vi "TupnOn.vi"(8 "error in (no error)":errorcluster, 11 "Pump_1AI_1DO_2DI in":refnum<class "Engine_1DO_2DI.lvclass">) -> (0 "error out":errorcluster, 3 "Pump_1AI_1DO_2DI out":refnum<class "Engine_1DO_2DI.lvclass">)   [LabVIEW 2019, in "Engine_1DO_2DI.lvclass"]
uses:
  Engine_1DO_2DI.lvclass
  C:/Users/H4001/Documents/GitHub/H4000/src/Device_class/Device.lvclass
  Engine_1DO_2DI.lvclass/Engine_1DO_2DI.ctl
  Device_class/Device.lvclass/Device.ctl
  TypeDef/State Engine.ctl
  FPGA_API_class/FPGA API.lvclass
  Device_class/Device.lvclass
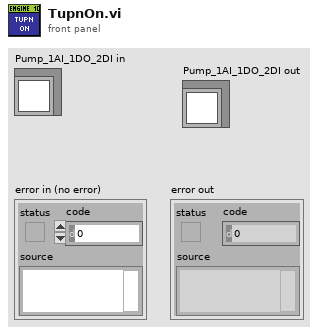
[diagram p1: front panel]
types:
  T1 = typedef "State Engine.ctl" = enum16{"Unknown", "Off", "TupningOn", "On", "TurningOff"}
  T2 = typedef "DO index.ctl" = u8
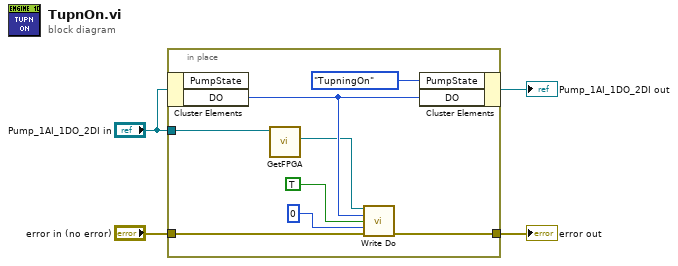
[diagram p0: block diagram]
diagram:
  n1 = in-place {
    in-place-border: [w8] -> w3
    in-place-border: "error in (no error)" -> [w7]
    in-place-border: "Pump_1AI_1DO_2DI in" -> [w6]
    n2 = in-place-cluster #1("Pump_1AI_1DO_2DI in") -> ("DO"=w10:T2)  [unwired: 1 out]
    n3 = call "GetFPGA.vi"("Device in"=w6) -> ("FPGA API.lvclass"=w5:refnum<class "FPGA API.lvclass">)  [unwired: 10 in]
    n4 = call "Write Do.vi"("FPGA API in"=w5, "#DO"=w10, "value"=TRUE, "Time uSec"=u32 0, "error in (no error)"=w7) -> ("error out"=w8:errorcluster)  [unwired: 9 in, 1 out]
    n5 = in-place-cluster #1("PumpState"=State_Engine."TupningOn", "DO"=w10) -> (→"Pump_1AI_1DO_2DI out":refnum<class "Engine_1DO_2DI.lvclass">)
  }
  "error out" <- w3
